vi "Updater Get Datafinder Name.vi"(8 "error in (no error)":errorcluster, 11 "spartan install dir":path) -> (0 "error out":errorcluster, 3 "datafinder name":string)   [LabVIEW 2011]
uses:
  <vilib>/Utility/config.llb/Read Key (String).vi
  <vilib>/Utility/config.llb/NI_LVConfig.lvlib
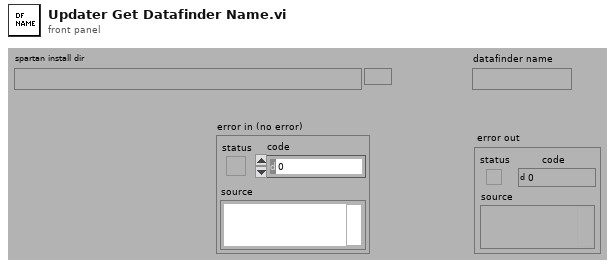
[diagram p1: front panel]
types:
  T1 = typedef "NI_LVConfig.lvlib/Config Data RefNum.ctl" = refnum<k1>
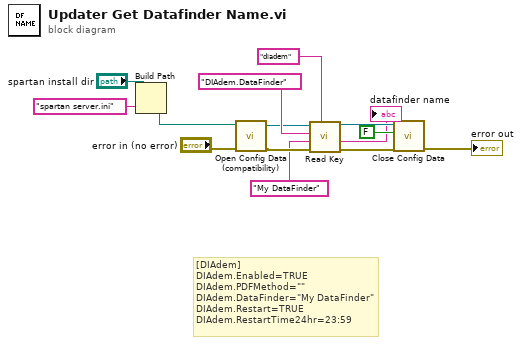
[diagram p0: block diagram]
diagram:
  # "[DIAdem]\nDIAdem.Enabled=TRUE\nDIAdem.PDFMethod=\"\"\nDIAdem.DataFinder=\"My DataFinder\"\nDIAdem.Restart=TRUE\nDIAdem.RestartTime24hr=23:59"
  n1 = Build Path(base path="spartan install dir", name or relative path="spartan server.ini") -> (appended path=w2:path)
  n2 = call <vilib>:"Open Config Data (compatibility).vi"("error in (no error)"="error in (no error)", "configuration file path"=w2) -> ("error out"=w14:errorcluster, "refnum"=w10:T1)  [unwired: 7 in, 1 out]
  n3 = call-poly <vilib>:"Read Key.vi"("section"="diadem", "error in (no error)"=w14, "default value"="My DataFinder" ("DataFinder (\"My DataFinder\")"), "key"="DIAdem.DataFinder", "refnum"=w10) -> ("error out"=w9:errorcluster, "value"=→"datafinder name":string, "refnum out"=w8:T1)  [unwired: 1 in, 3 out]
  n4 = call <vilib>:"Close Config Data.vi"("error in (no error)"=w9, "write file if changed (T)"=FALSE ("write configuration file? (T)"), "refnum"=w8) -> ("error out"=→"error out":errorcluster)  [unwired: 8 out]
